vi "Decorations - Set Tag.vi"(8 "error in (no error)":errorcluster) -> (0 "error out":errorcluster)   [LabVIEW 2017]
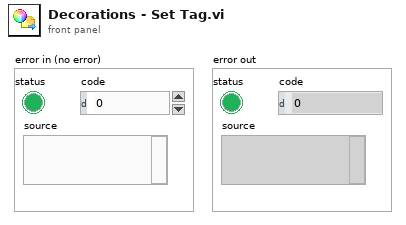
[diagram p1: front panel]
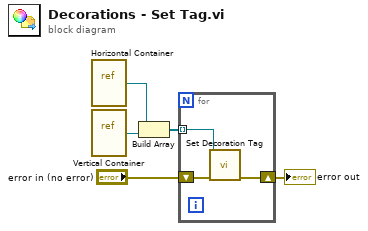
[diagram p0: block diagram]
diagram:
  n1 = vi-ref "Horizontal Container.vi"() -> (w5:refnum<vi>)
  n2 = vi-ref "Vertical Container.vi"() -> (w4:refnum<vi>)
  n3 = Build Array(w5, w4) -> (w3:refnum<vi>[])
  n4 = for {
    tunnel: w3 -> [w8] mode=indexing
    shift-right: [w7] -> w1
    shift-left: "error in (no error)" -> [w6]
    n5 = call "Set Decoration Tag.vi"("error in (no error)"=w6, "VI Refnum"=w8) -> ("error out"=w7:errorcluster)  [unwired: 9 in]
  }
  "error out" <- w1
